vi "robotconstants.vi"() -> ()   [LabVIEW 2020]
panel:
  out "Cowl_Gear_Ratio":dbl
  out "Shooter_Upper_Wheel_Diameter (in)":dbl
  out "Shooter_Lower_Wheel_Diameter (in)":dbl
  out "Turret_Gear_Ratio":dbl
  out "Azimuth_Gear_Ratio":dbl
  out "Drive_High_Gear_Ratio":dbl
  out "Drive_Low_Gear_Ratio":dbl
  out "Drive_Wheel_Diameter (in)":dbl
  out "Robot_Width_Bumpers (in)":dbl
  out "Robot_Length_Bumpers (in)":dbl
  out "Cowl_Max_Extension_Position (deg)":dbl
  out "Cowl_Homing_Position (deg)":dbl
  out "Turret_Homing_Position (deg)":dbl
  out "Turret_Center_Y (in)":dbl
  out "Turret_Center_X (in)":dbl
  out "Turret_Radius (in)":dbl
  out "Robot_Minimum_Dimension (in)":dbl
  out "Robot_Width (in)":dbl
  out "Robot_Length (in)":dbl
  out "Angle_from_LL_to_Horizontal (deg)":dbl
  out "Height_from_LL_To_Ground_(in)":dbl
  out "Legal_Shooter_Setpoints":string[](array[string])
  out "Legal_Actuator_Names":string[](array[string])
  out "Legal_Drivers":string[](array[string])
  out "Legal_Auto_Plays":string[](array[string])
  out "Max_Robot_Ground_Speed_(ft/s)":dbl
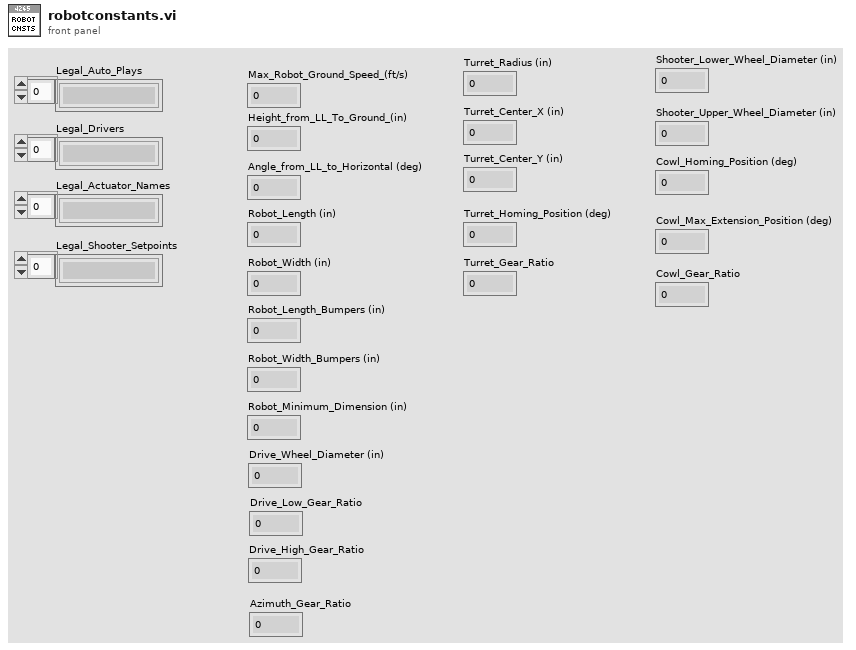
[diagram p1: front panel]
diagram:
